vi "__uintSetBase.vi"(8 "Error in (no error)":errorcluster, 10 "Base (decimal)":T1=10 items=["Binary"=2, "Octal"=8, "Decimal"=10, "Hexadecimal"=16, "Hexatrigesimal"=36, "ASCII"=64], 11 "Uint in":refnum<class "UintClass.lvclass">) -> (0 "Error out":errorcluster, 3 "Uint out":refnum<class "UintClass.lvclass">)   [LabVIEW 2011, in "UintClass.lvclass"]
uses:
  UintClass.lvclass
  enumBase.ctl
  UintClass.lvclass/UintClass.ctl
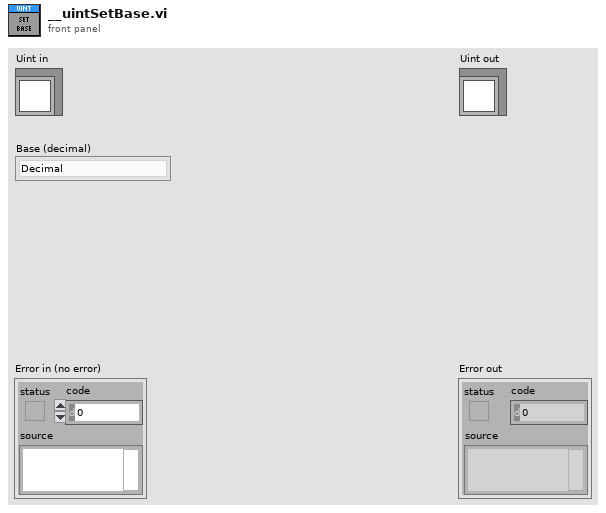
[diagram p1: front panel]
types:
  T1 = typedef "UintClass.lvclass/enumBase.ctl" = u16
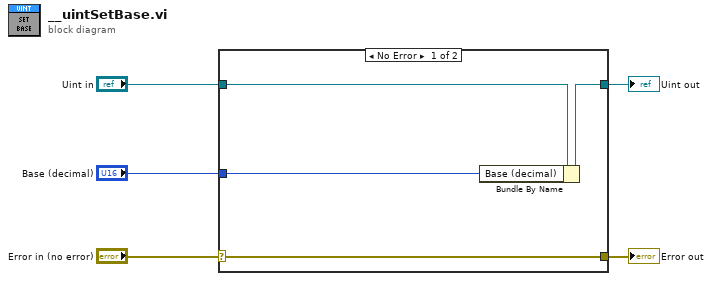
[diagram p0: block diagram]
diagram:
  n1 = case shown="No Error" "Error in (no error)" {
    selector: "Error in (no error)" -> [w9 w10]
    tunnel: [w9 w10] -> w4
    tunnel: [w7 w11] -> w2
    tunnel: "Uint in" -> [w8 w11]
    tunnel: "Base (decimal)" -> [w6 _]
    frame No Error {
      n2 = Bundle By Name(cluster=w8, "Base (decimal)"=w6) -> (w7:refnum<class "UintClass.lvclass">)
    }
    frame Error {
    }
  }
  "Error out" <- w4
  "Uint out" <- w2
